vi "BRig_dataMTrig_Loop_c.vi"() -> (2 "output_Loop_c":i32)   [LabVIEW 2014]
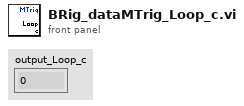
[diagram p1: front panel]
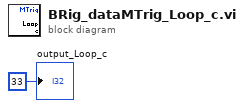
[diagram p0: block diagram]
diagram:
  "output_Loop_c" <- 33 ("output_iBlock")
